vi "Generate HPPC Plots.vi"(8 "error in (no error)":errorcluster, 10 "HPPC Parameters":T1={"HPPC Mode"=1, "Pulse Duration (S)"=10.0, "Charge Current (A)"=25.0, "Rest Duration (S)"=10.0, "Discharge Current (A)"=25.0, "Temperature (C)"=25.0, "Nominal Capacity (Ah)"=10.0, "Initial SoC (%)"=100.0, "Final SoC (%)"=50.0, "SoC Interval (%)"=10.0, "SoC Step Current (A)"=100.0, "SoC Step Relax (S)"=10.0} {"HPPC Mode" items=["Discharge Only", "Full Cycle"]; "Nominal Capacity (Ah)" min=0.0 max=100.0; "Final SoC (%)" min=0.0 max=100.0; "SoC Interval (%)" min=0.0 max=100.0; "Initial SoC (%)" min=0.0 max=100.0}, 11 "TDMS Data File":path) -> (0 "error out":errorcluster, 2 "HPPC Power":cluster{dbl[], dbl[]}(graph), 3 "HPPC Voltage":cluster{dbl[], dbl[]}(graph))   [LabVIEW 2023, in "DCIR_HPPC.lvclass"]
uses:
  DCIR_HPPC.lvclass
  HPPC Parameters.ctl
  HPPC Mode.ctl
  DCIR_HPPC.lvclass/DCIR_HPPC.ctl
panel:
  out "measured voltage":dbl[][](array[numeric])
  out "measured current":dbl[][](array[numeric])
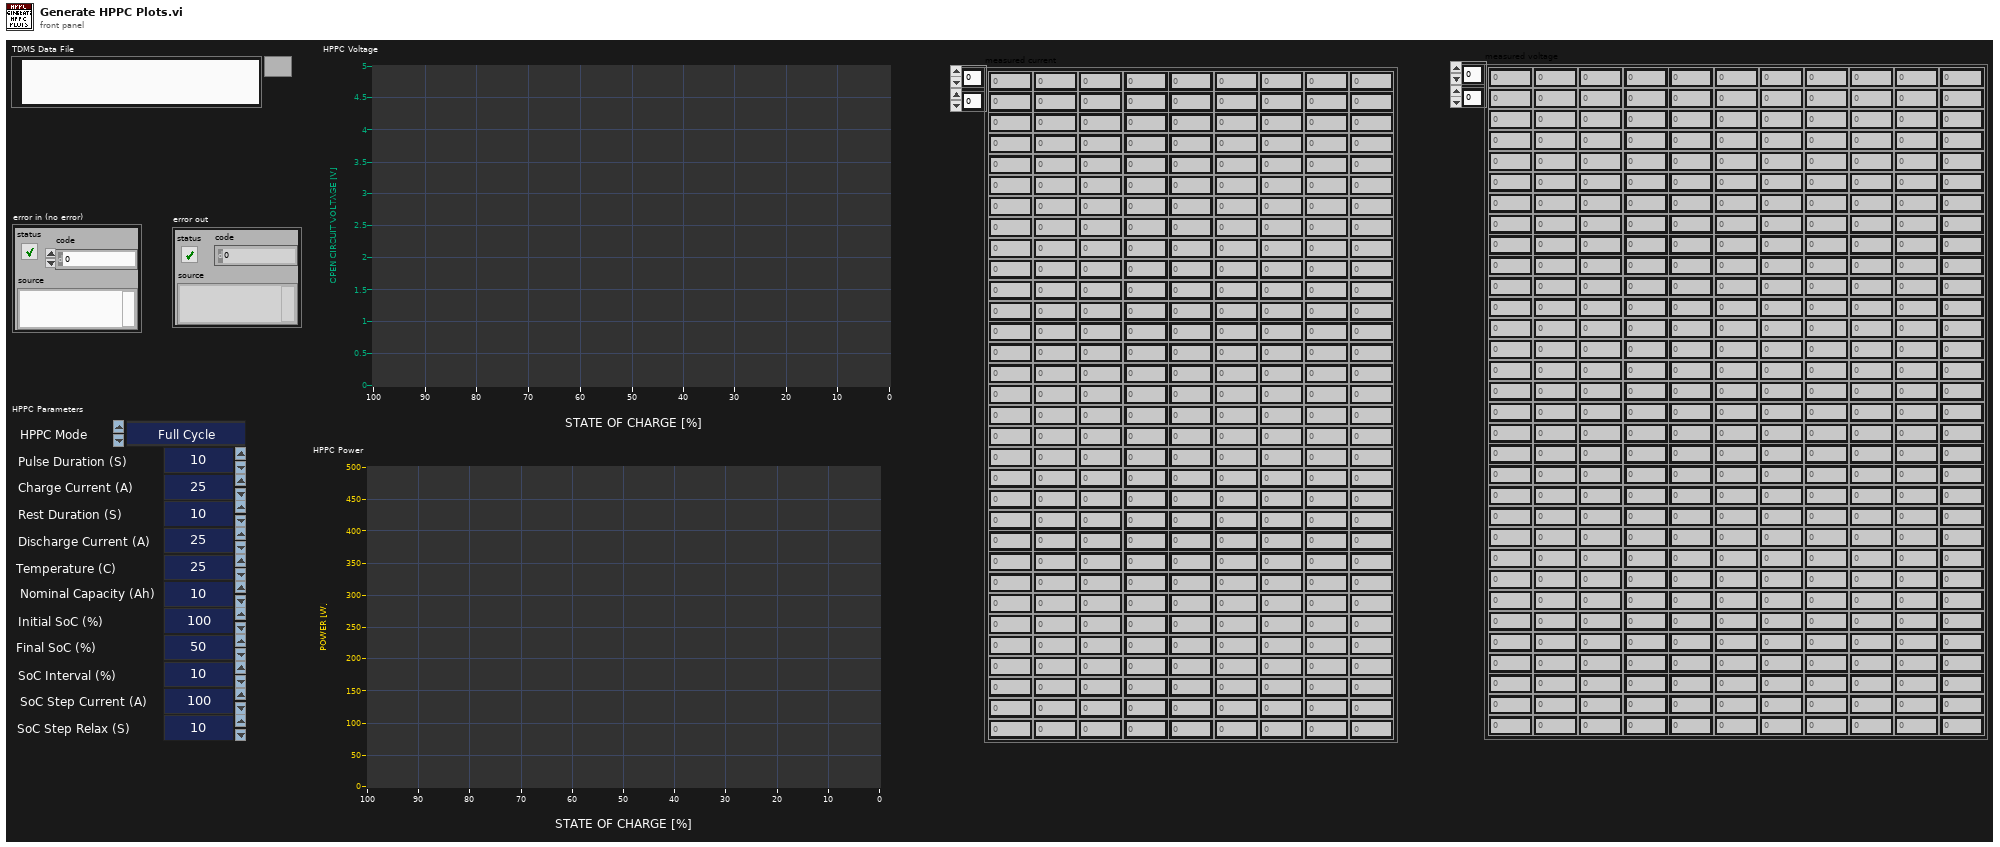
[diagram p1: front panel]
types:
  T1 = typedef "DCIR_HPPC.lvclass/HPPC Parameters.ctl" = cluster{"HPPC Mode":T2, "Pulse Duration (S)":dbl, "Charge Current (A)":dbl, "Rest Duration (S)":dbl, "Discharge Current (A)":dbl, "Temperature (C)":dbl, "Nominal Capacity (Ah)":dbl, "Initial SoC (%)":dbl, "Final SoC (%)":dbl, "SoC Interval (%)":dbl, "SoC Step Current (A)":dbl, "SoC Step Relax (S)":dbl}
  T2 = typedef "DCIR_HPPC.lvclass/HPPC Mode.ctl" = u16
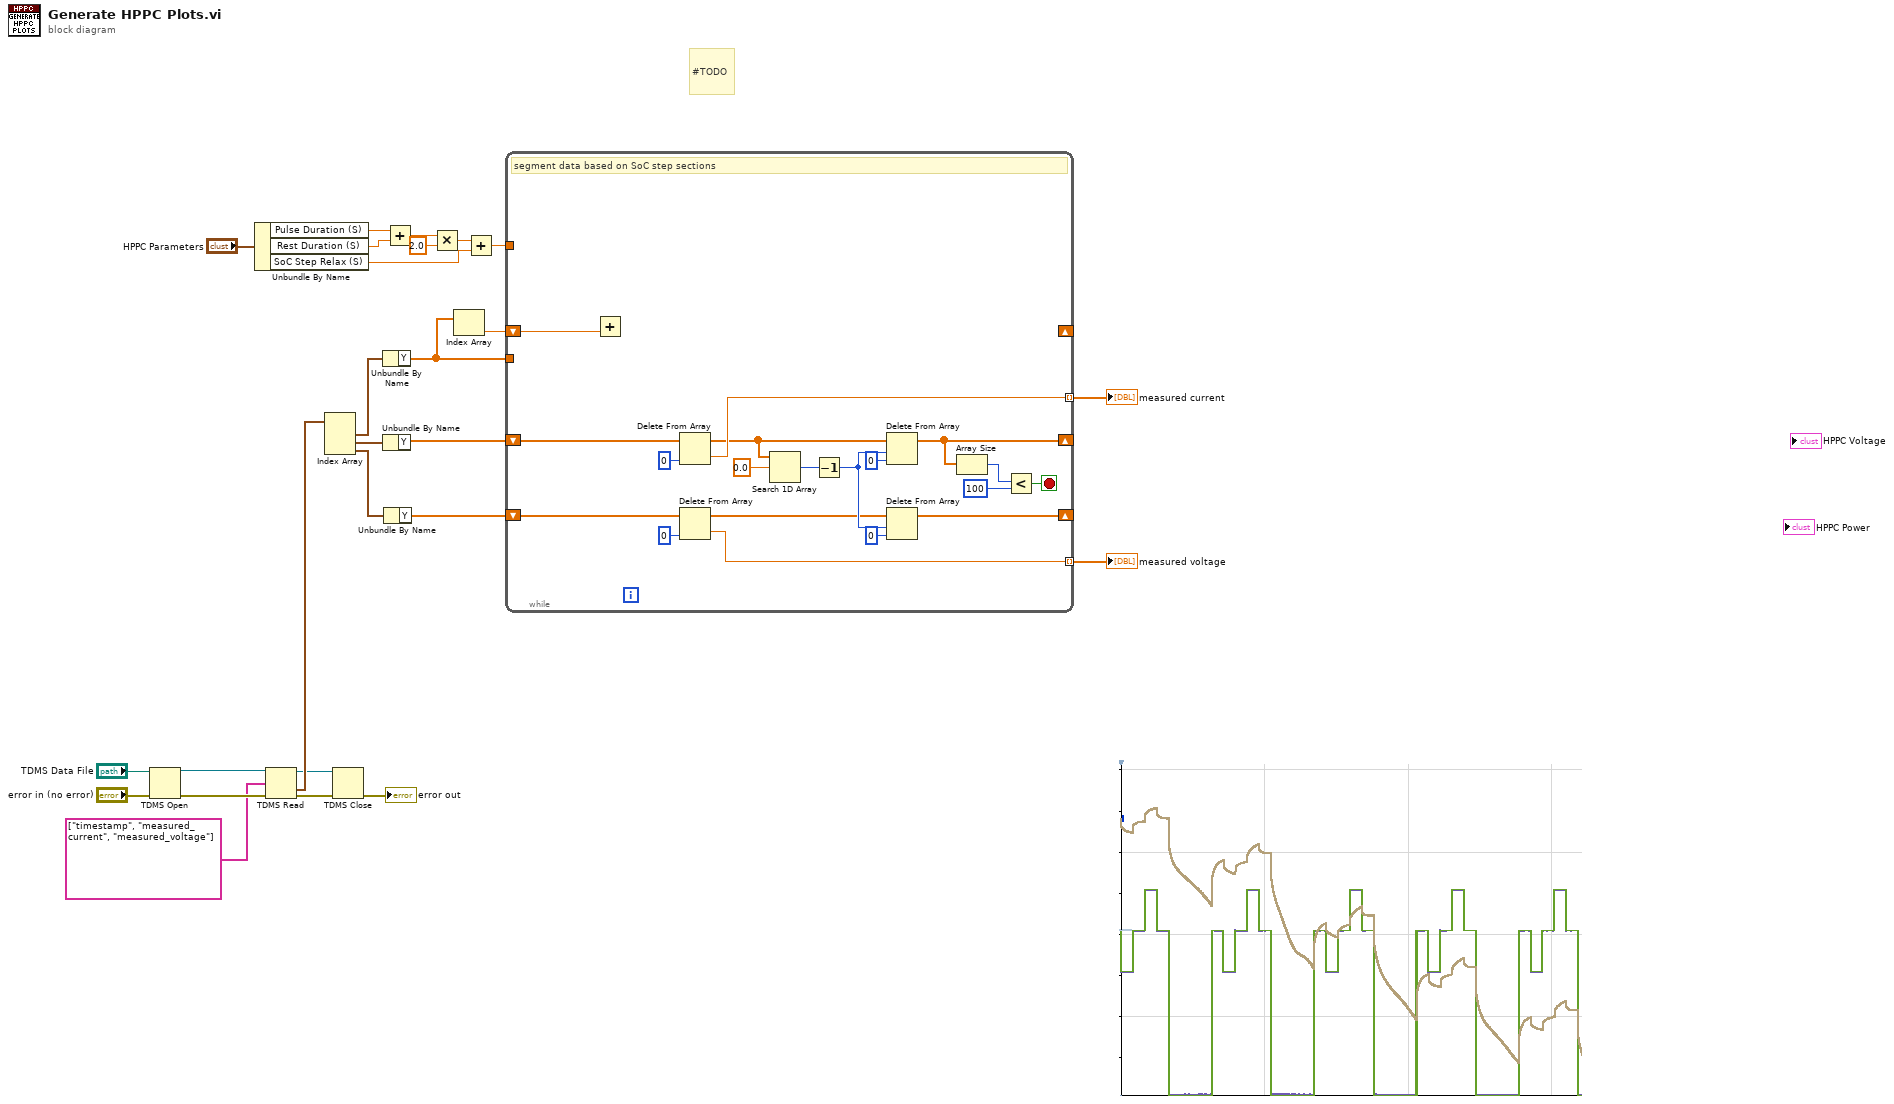
[diagram p0: block diagram]
diagram:
  # "#TODO"
  n1 = TDMS Open(8:"error in (no error)", 11:"TDMS Data File") -> (0:w24:errorcluster, 3:w23:refnum<k34>)  [unwired: 5 in]
  n2 = Unbundle By Name("HPPC Parameters") -> ("Pulse Duration (S)"=w12:dbl, "Rest Duration (S)"=w11:dbl, "SoC Step Relax (S)"=w7:dbl)
  n3 = TDMS Read(0:w23, 7:string[] ["timestamp", "measured_current", "measured_voltage"] ("channel name(s) in"), 11:w24) -> (4:w19:refnum<k34>, 10:w21:waveform(dbl)[], 15:w20:errorcluster)  [unwired: 5 in, 3 out]
  n4 = Index Array(array=w21) -> (element #1=w4:waveform(dbl), element #2=w16:waveform(dbl), element #3=w17:waveform(dbl))  [unwired: 3 in]
  n5 = TDMS Close(8:w20, 11:w19) -> (0:→"error out":errorcluster)  [unwired: 1 out]
  n6 = Unbundle By Name(w4) -> ("Y"=w3:dbl[])
  n7 = Unbundle By Name(w16) -> ("Y"=w14:dbl[])
  n8 = Unbundle By Name(w17) -> ("Y"=w13:dbl[])
  n9 = Add(x=w12, y=w11) -> (x+y=w10:dbl)
  n10 = Multiply(x=w10, y=2.0) -> (x*y=w8:dbl)
  n11 = Index Array(array=w3) -> (element=w1:dbl)  [unwired: 1 in]
  n12 = Add(x=w8, y=w7) -> (x+y=w2:dbl)
  n13 = while {
    shift-right: [w38] -> _
    shift-left: w14 -> [w45]
    shift-right: [w30] -> _
    shift-left: w13 -> [w44]
    tunnel: [w40] -> w6 mode=indexing
    tunnel: [w39] -> w5 mode=indexing
    tunnel: w3 -> [_]
    tunnel: w2 -> [_]
    shift-right: _ -> [_]
    shift-left: w1 -> [w27]
    stop <- w43 stop-if-true
    # "segment data based on SoC step sections"
    n14 = Add(y=w27) -> ()  [unwired: 1 in, 1 out]
    n15 = Delete From Array(array=w45, index=0) -> (deleted portion=w40:dbl, array with subset deleted=w35:dbl[])  [unwired: 1 in]
    n16 = Delete From Array(array=w44, index=0) -> (deleted portion=w39:dbl, array with subset deleted=w31:dbl[])  [unwired: 1 in]
    n17 = Search 1D Array(1D array=w35, element=0.0) -> (index of element=w36:i32)  [unwired: 1 in]
    n18 = Decrement(x=w36) -> (x-1=w33:i32)
    n19 = Delete From Array(array=w35, length=w33, index=0) -> (array with subset deleted=w38:dbl[])  [unwired: 1 out]
    n20 = Delete From Array(array=w31, length=w33, index=0) -> (array with subset deleted=w30:dbl[])  [unwired: 1 out]
    n21 = Array Size(array=w38) -> (size(s)=w28:i32)
    n22 = Less?(x=w28, y=100 ("x")) -> (x < y?=w43:bool)
  }
  "measured current" <- w6
  "measured voltage" <- w5
